vi "Ex3.vi"() -> ()   [LabVIEW 2012]
doc: "Example VI: reads in states of the buttons on Baxter's arm"
uses:
  <userlib>/ROSforLV/ROS/Code/SubVIs/BaxterButtons.ctl
  <userlib>/ROSforLV/ROS/Code/SubVIs/DigitalIOComponents.ctl
panel:
  in  "stop":bool
  out "Left ITB":T1
  # "Hitting the long buttons on his wrist toggles the lights on his arms"
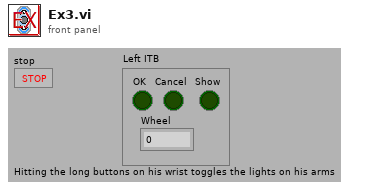
[diagram p1: front panel]
types:
  T1 = cluster{"OK":bool, "Cancel":bool, "Show":bool, "Wheel":u8}
  T2 = typedef "BaxterButtons.ctl" = enum16{"left_itb", "right_itb", "torso_left_itb", "torso_right_itb"}
  T3 = typedef "DigitalIOComponents.ctl" = enum16{"left_lower_cuff", "right_lower_cuff", "left_lower_button", "right_lower_button", "left_upper_button", "right_upper_button", "left_shoulder_button", "right_shoulder_button"}
  T4 = cluster{"Component":T3, "state":i8, "is input only":bool}[]
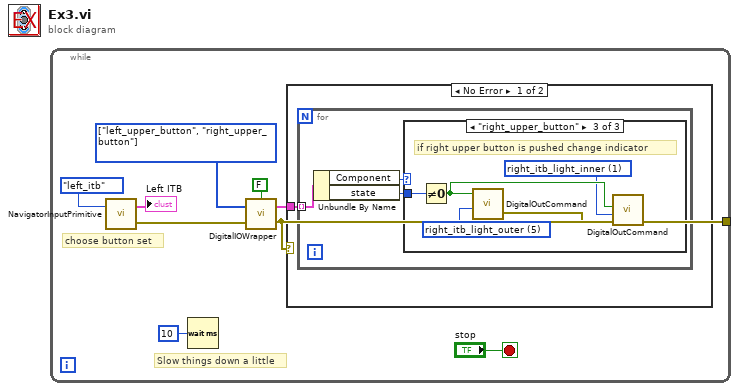
[diagram p0: block diagram]
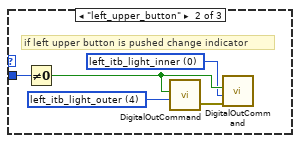
[diagram p3: hidden frame]
diagram:
  n1 = while {
    tunnel: [w2] -> _
    stop <- "stop" stop-if-true
    w4 = T3[] [enum."left_upper_button", enum."right_upper_button"] items=["left_lower_cuff", "right_lower_cuff", "left_lower_button", "right_lower_button", "left_upper_button", "right_upper_button", "left_shoulder_button", "right_shoulder_button"] ("Component IDs")
    # "choose button set"
    # "Slow things down a little"
    n2 = call <userlib>:"NavigatorInputPrimitive.vi"("Component"=BaxterButtons."left_itb") -> ("error out"=w5:errorcluster, "Navigator Inputs"=→"Left ITB":T1)  [unwired: 2 in]
    n3 = Wait (ms)(milliseconds to wait=u32 10) -> ()  [unwired: 1 out]
    n4 = call <userlib>:"DigitalIOWrapper.vi"("error in"=w5, "Component IDs"=w4, "True Only (T)"=FALSE) -> ("error out"=w2:errorcluster, "Changed_IO"=w3:T4)
    n5 = case shown="No Error" w2 {
      tunnel: w3 -> [w10 _]
      frame No Error {
        n6 = for {
          tunnel: w10 -> [w13] mode=indexing
          n7 = Unbundle By Name(w13) -> ("Component"=w12:T3, "state"=w11:i8)
          n8 = case shown="\"right_upper_button\"" w12 {
            tunnel: w11 -> [_ w18 w23]
            frame Default {
            }
            frame "left_upper_button" {
              w14 = u16 0 items=["left_itb_light_inner", "right_itb_light_inner", "torso_left_itb_light_inner", "torso_right_itb_light_inner", "left_itb_light_outer", "right_itb_light_outer", "torso_left_itb_light_outer", "torso_right_itb_light_outer", ""] ("Component ID")
              w17 = u16 4 items=["left_itb_light_inner", "right_itb_light_inner", "torso_left_itb_light_inner", "torso_right_itb_light_inner", "left_itb_light_outer", "right_itb_light_outer", "torso_left_itb_light_outer", "torso_right_itb_light_outer", ""] ("Component ID")
              # "if left upper button is pushed change indicator"
              n9 = Not Equal To 0?(x=w18) -> (x != 0?=w15:bool)
              n10 = call <userlib>:"DigitalOutCommand.vi"("Component ID"=w17, "State"=w15) -> ("error out"=w16:errorcluster)  [unwired: 3 in]
              n11 = call <userlib>:"DigitalOutCommand.vi"("error in"=w16, "Component ID"=w14, "State"=w15) -> ()  [unwired: 2 in, 1 out]
            }
            frame "right_upper_button" {
              w20 = u16 1 items=["left_itb_light_inner", "right_itb_light_inner", "torso_left_itb_light_inner", "torso_right_itb_light_inner", "left_itb_light_outer", "right_itb_light_outer", "torso_left_itb_light_outer", "torso_right_itb_light_outer", ""] ("Component ID")
              w22 = u16 5 items=["left_itb_light_inner", "right_itb_light_inner", "torso_left_itb_light_inner", "torso_right_itb_light_inner", "left_itb_light_outer", "right_itb_light_outer", "torso_left_itb_light_outer", "torso_right_itb_light_outer", ""] ("Component ID")
              # "if right upper button is pushed change indicator"
              n12 = Not Equal To 0?(x=w23) -> (x != 0?=w21:bool)
              n13 = call <userlib>:"DigitalOutCommand.vi"("Component ID"=w22, "State"=w21) -> ("error out"=w19:errorcluster)  [unwired: 3 in]
              n14 = call <userlib>:"DigitalOutCommand.vi"("error in"=w19, "Component ID"=w20, "State"=w21) -> ()  [unwired: 2 in, 1 out]
            }
          }
        }
      }
      frame Error {
      }
    }
  }
